vi "Experiment4TimeDelay.vi"() -> ()   [LabVIEW 2016]
uses:
  Other Models/EFD Ultimus V/EFD Ultimus V.lvlib
panel:
  out "Comm Out":string
  in  "Comm In":string
  in  "Serial Configuration":T1={"Baud Rate "=115200, "Parity "=0, "Data Bits "=8, "Stop Bits"=10} {"Stop Bits" items=["1.0"=10, "1.5"=15, "2.0"=20]; "Data Bits" items=["7"=7, "8"=8]; "Parity" items=["None", "Odd", "Even"]; "Baud Rate" items=["9600"=9600, "19200"=19200, "38400"=38400, "115200"=115200]}
  in  "VISA resource name":refnum<visa-resource-name>="COM1"
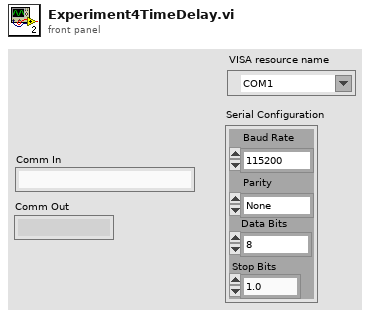
[diagram p1: front panel]
types:
  T1 = cluster{"Baud Rate ":u32, "Parity ":u16, "Data Bits ":u16, "Stop Bits":u16}
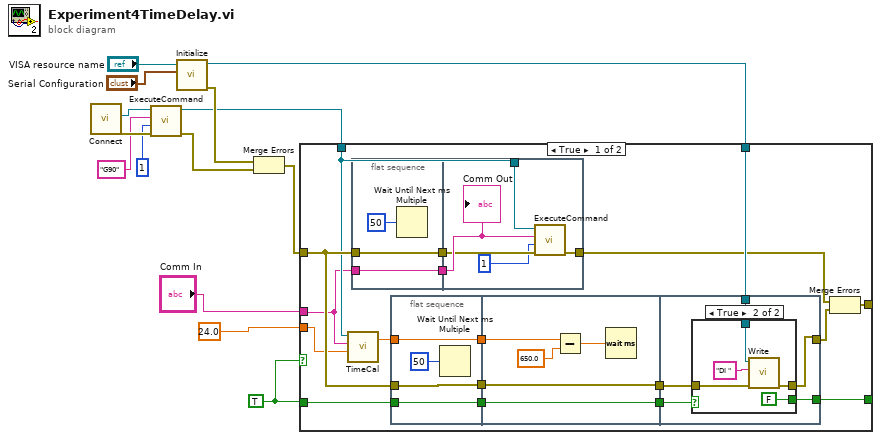
[diagram p0: block diagram]
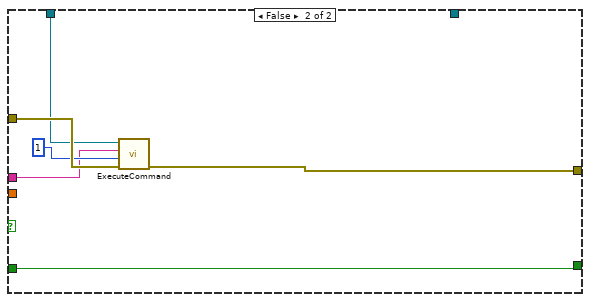
[diagram p3: hidden frame]
diagram:
  w9 = TRUE
  n1 = call "Connect.vi"() -> ("error out"=w5:errorcluster, "controller"=w6:refnum<k24>)  [unwired: 10 in]
  n2 = call "ExecuteCommand.vi"("error in (no error)"=w5, "taskId"=1, "Command Code"="G90", "controller in"=w6) -> ("error out"=w4:errorcluster, "controller out"=w3:refnum<k24>)  [unwired: 5 in, 1 out]
  n3 = call "Initialize.vi"("Serial Configuration"="Serial Configuration", "VISA resource name"="VISA resource name") -> ("error out"=w11:errorcluster, "VISA resource name out"=w12:refnum<visa-resource-name>)  [unwired: 8 in]
  n4 = Merge Errors(w11, w4) -> (w10:errorcluster)
  n5 = case shown="True" w9 {
    tunnel: w10 -> [w24 w67]
    tunnel: [w22 w66] -> _
    tunnel: w3 -> [w17 w64]
    tunnel: "Comm In" -> [w16 w63]
    tunnel: w12 -> [w30 _]
    tunnel: w9 -> [w32 w62]
    tunnel: [w31 w62] -> _
    tunnel: 24.0 -> [w15 _]
    frame True {
      n6 = call "TimeCal.vi"("Speed In"=w15, "Command"=w16, "controller in"=w17) -> ("Time(ms)"=w18:dbl)  [unwired: 7 in, 1 out]
      n7 = flat-sequence {
        tunnel: w16 -> [w55]
        tunnel: [w55] -> w25
        tunnel: w24 -> [w54]
        tunnel: [w54] -> w23
        tunnel: w25 -> [w61]
        tunnel: w23 -> [w60]
        tunnel: [w59] -> w20
        tunnel: w17 -> [w58]
        frame #0 {
          n8 = Wait Until Next ms Multiple(millisecond multiple=50) -> ()  [unwired: 1 out]
        }
        frame #1 {
          n9 = call "ExecuteCommand.vi"("error in (no error)"=w60, "taskId"=1, "Command Code"=w61, "controller in"=w58) -> ("error out"=w59:errorcluster)  [unwired: 5 in, 2 out]
          "Comm Out" <- w61
        }
      }
      n10 = flat-sequence {
        tunnel: w32 -> [w36]
        tunnel: [w36] -> w28
        tunnel: [w34] -> w27
        tunnel: w24 -> [w34]
        tunnel: w18 -> [w33]
        tunnel: [w33] -> w19
        tunnel: [w41] -> w29
        tunnel: w28 -> [w41]
        tunnel: w27 -> [w40]
        tunnel: [w40] -> w26
        tunnel: w19 -> [w39]
        tunnel: [w45] -> w31
        tunnel: [w44] -> w21
        tunnel: w30 -> [w43]
        tunnel: w29 -> [w46]
        tunnel: w26 -> [w42]
        frame #0 {
          n11 = Wait Until Next ms Multiple(millisecond multiple=50) -> ()  [unwired: 1 out]
        }
        frame #1 {
          n12 = Subtract(x=w39, y=650.0) -> (x-y=w38:dbl)
          n13 = Wait (ms)(milliseconds to wait=w38) -> ()  [unwired: 1 out]
        }
        frame #2 {
          n14 = case shown="True" w46 {
            selector: w46 -> [w47 _]
            tunnel: w42 -> [w48 w52]
            tunnel: [w48 w51] -> w44
            tunnel: [w47 FALSE] -> w45
            tunnel: w43 -> [_ w50]
            frame False {
            }
            frame True {
              n15 = call "Write.vi"("error in (no error)"=w52, "Command To Write"="DI ", "VISA resource name"=w50) -> ("error out"=w51:errorcluster)  [unwired: 7 in, 1 out]
            }
          }
        }
      }
      n16 = Merge Errors(w20, w21) -> (w22:errorcluster)
    }
    frame False {
      n17 = call "ExecuteCommand.vi"("error in (no error)"=w67, "taskId"=1, "Command Code"=w63, "controller in"=w64) -> ("error out"=w66:errorcluster)  [unwired: 5 in, 2 out]
    }
  }
